vi "RichToFlatcif_management_common_MonitorU64.vi"(5 "OutputClusterType":T1, 11 "InputCluster":T2) -> (3 "OutputCluster":T1)   [LabVIEW 2021, in "CIFCorePlugin_server.lvlib"]
uses:
  CIFCorePlugin_server.lvlib
  cif_management_common_MonitorU64.ctl
  cif_management_common_MonitorU64_Flat.ctl
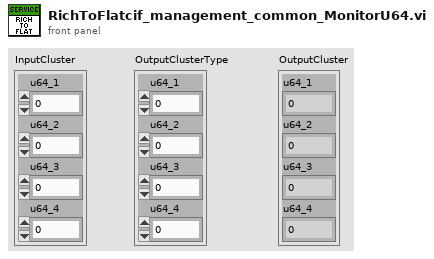
[diagram p1: front panel]
types:
  T1 = typedef "CIFCorePlugin_server.lvlib/cif_management_common_MonitorU64_Flat.ctl" = cluster{"u64_1":u64, "u64_2":u64, "u64_3":u64, "u64_4":u64}
  T2 = typedef "CIFCorePlugin_server.lvlib/cif_management_common_MonitorU64.ctl" = cluster{"u64_1":u64, "u64_2":u64, "u64_3":u64, "u64_4":u64}
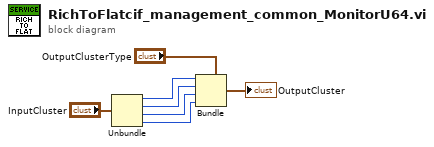
[diagram p0: block diagram]
diagram:
  n1 = Unbundle "Unbundle"("InputCluster") -> ("u64_1"=w4:u64, "u64_2"=w3:u64, "u64_3"=w2:u64, "u64_4"=w1:u64)
  n2 = Bundle "Bundle"(cluster="OutputClusterType", "u64_1"=w4, "u64_2"=w3, "u64_3"=w2, "u64_4"=w1) -> (→"OutputCluster":T1)
